vi "TimingBlocks.vi"() -> ()   [LabVIEW 2020]
panel:
  out "date/time string":string
  out "time string":string
  out "current time":timestamp
  out "relative seconds":dbl format="%_19f"
  out "millisecond timer value":u32
  in  "milliseconds to wait":u32
  in  "stop":bool
  out "Numeric":i32
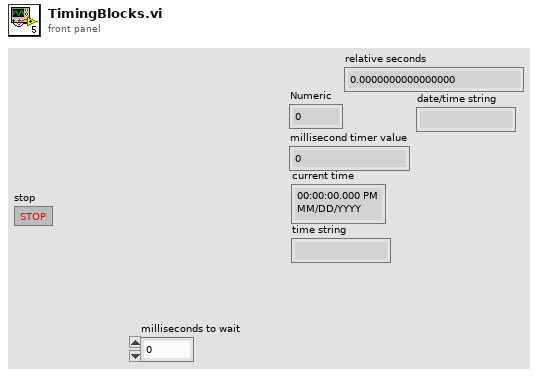
[diagram p1: front panel]
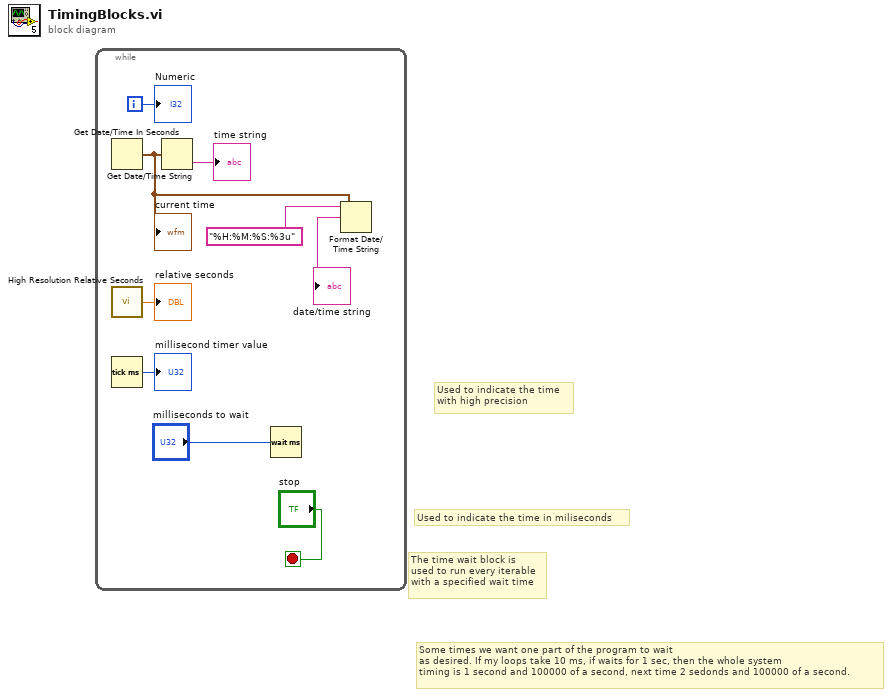
[diagram p0: block diagram]
diagram:
  # "Used to indicate the time \nwith high precision"
  # "Used to indicate the time in miliseconds"
  # "Some times we want one part of the program to wait \nas desired. If my loops take 10 ms, if waits for 1 sec, then the whole system\ntiming is 1 second and 100000 of a second, next time 2 sedonds and 100000 of a second."
  # "The time wait block is\nused to run every iterable\nwith a specified wait time"
  n1 = while {
    i -> [w9]
    stop <- "stop" stop-if-true
    n2 = Get Date/Time In Seconds() -> (seconds since 1Jan1904=w3:timestamp)
    "current time" <- w3
    n3 = call <vilib>:"High Resolution Relative Seconds.vi"() -> ("relative seconds"=→"relative seconds":dbl)
    n4 = Tick Count (ms)() -> (millisecond timer value=→"millisecond timer value":u32)
    n5 = Get Date/Time String(seconds (now)=w3) -> (time string=→"time string":string)  [unwired: 2 in, 1 out]
    n6 = Wait (ms)(milliseconds to wait="milliseconds to wait") -> ()  [unwired: 1 out]
    n7 = Format Date/Time String(time format string (%c)="%H:%M:%S:%3u", seconds (now)=w3) -> (date/time string=→"date/time string":string)  [unwired: 1 in]
    "Numeric" <- w9
  }
